vi "CV10.vi"() -> ()   [LabVIEW 2016]
uses:
  <vilib>/Analysis/baseanly.llb/Mean (DBL).vi
  <vilib>/DAQmx/read.llb/DAQmx Read (Analog 2D DBL NChan NSamp).vi
  <vilib>/DAQmx/create/channels.llb/DAQmx Create Channel (AI-Voltage-Basic).vi
  <vilib>/DAQmx/configure/timing.llb/DAQmx Timing (Sample Clock).vi
  <vilib>/DAQmx/miscellaneous.llb/DAQmx Fill In Error Info.vi
  <vilib>/imath/engines/lvmath2/RunTimeEngine/Managers/WorkSpace/UID Generator.vi
  <vilib>/imath/engines/lvmath2/RunTimeEngine/RunTimeType/NIMS_RunTimeType_From StrictType (excl LVString).vi
  <instcachedir>/0/NIMS_RunTimeType_From StrictType (excl LVString)_CEE1C65A8F1B491DB327E5E54E5E7674.lvgen/NIMS_RunTimeType_From StrictType (excl LVString)_CEE1C65A8F1B491DB327E5E54E5E7674_000.vi
  <vilib>/imath/engines/lvmath2/RunTimeEngine/LocalVariableDefStatement/MC_LocalVariableDefStatement_Display.vi
  <vilib>/imath/engines/lvmath2/RunTimeEngine/Managers/SymbolTable/Clear UID.vi
  <vilib>/imath/engines/lvmath2/RunTimeEngine/NodeEndStatement/NIMS_NodeEndStatement_Output.vi
  <instcachedir>/0/NIMS_NodeEndStatement_Output_53EC0D466D134D7ABD903AC30B43404B.lvgen/NIMS_NodeEndStatement_Output_53EC0D466D134D7ABD903AC30B43404B_009.vi
  <vilib>/imath/engines/lvmath2/RunTimeEngine/ErrorHandling/NIMS_Finalize Error.vi
  <vilib>/Analysis/NI_AALBase.lvlib
  <vilib>/imath/engines/lvmath2/RunTimeEngine/Managers/SymbolTable/NIMS_WorkSpace.lvlib
panel:
  out "Effective Sample Rate (Hz)":dbl=10.0
  in  "Display Length (s)":dbl=280.0 format="%#.3f"
  out "Time Step (ms)":dbl=100.0
  out "I-t":cluster{dbl[], dbl[]}(graph)
  in  "Samples to Average":i32=30000
  out "Elements in Queue":i32
  in  "Stop":bool
  in  "file path (use dialog), Create or Replace":path
  in  "Gain (mV/pA)":dbl=1.0
  out "I-V":cluster{dbl[], dbl[]}(graph)
  in  "Sampling Rate (Hz)":dbl=300000.0 format="%0.0f"
  in  "Voltage/Current Input Channels":tag="Dev1/ai0:1"
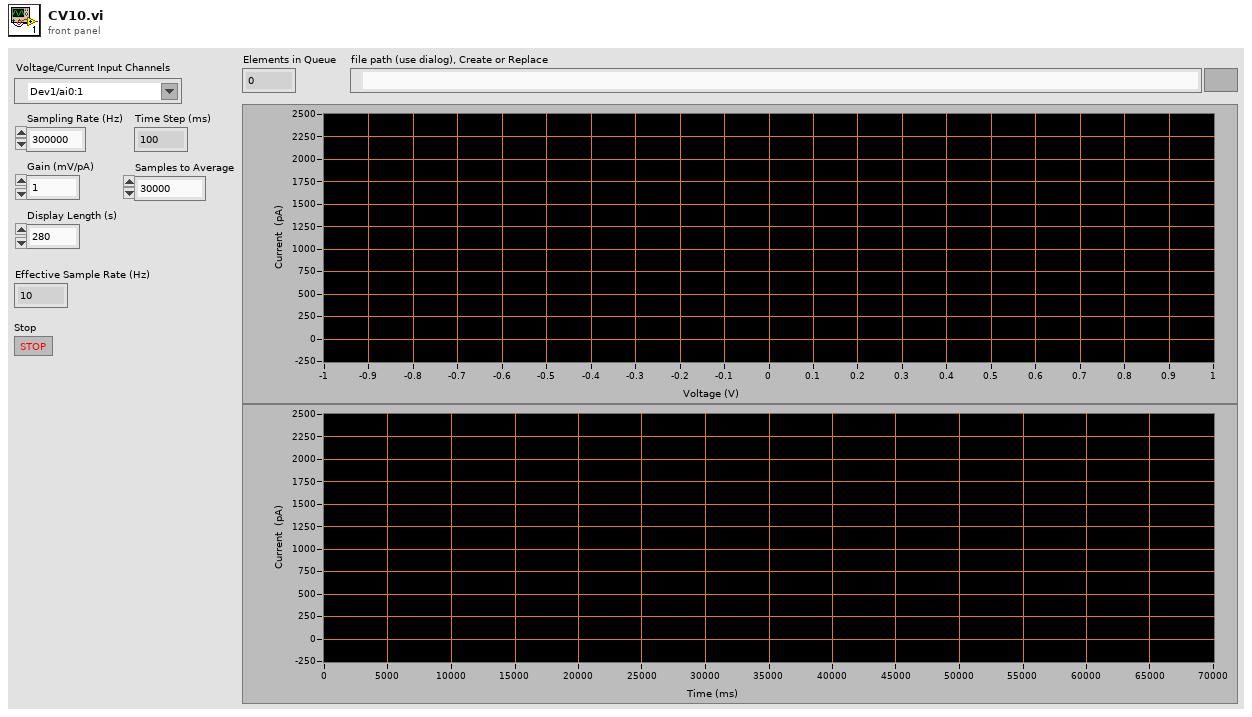
[diagram p1: front panel]
types:
  T1 = enum16{"open", "replace", "create", "open or create", "replace or create", "replace or create with confirmation"}
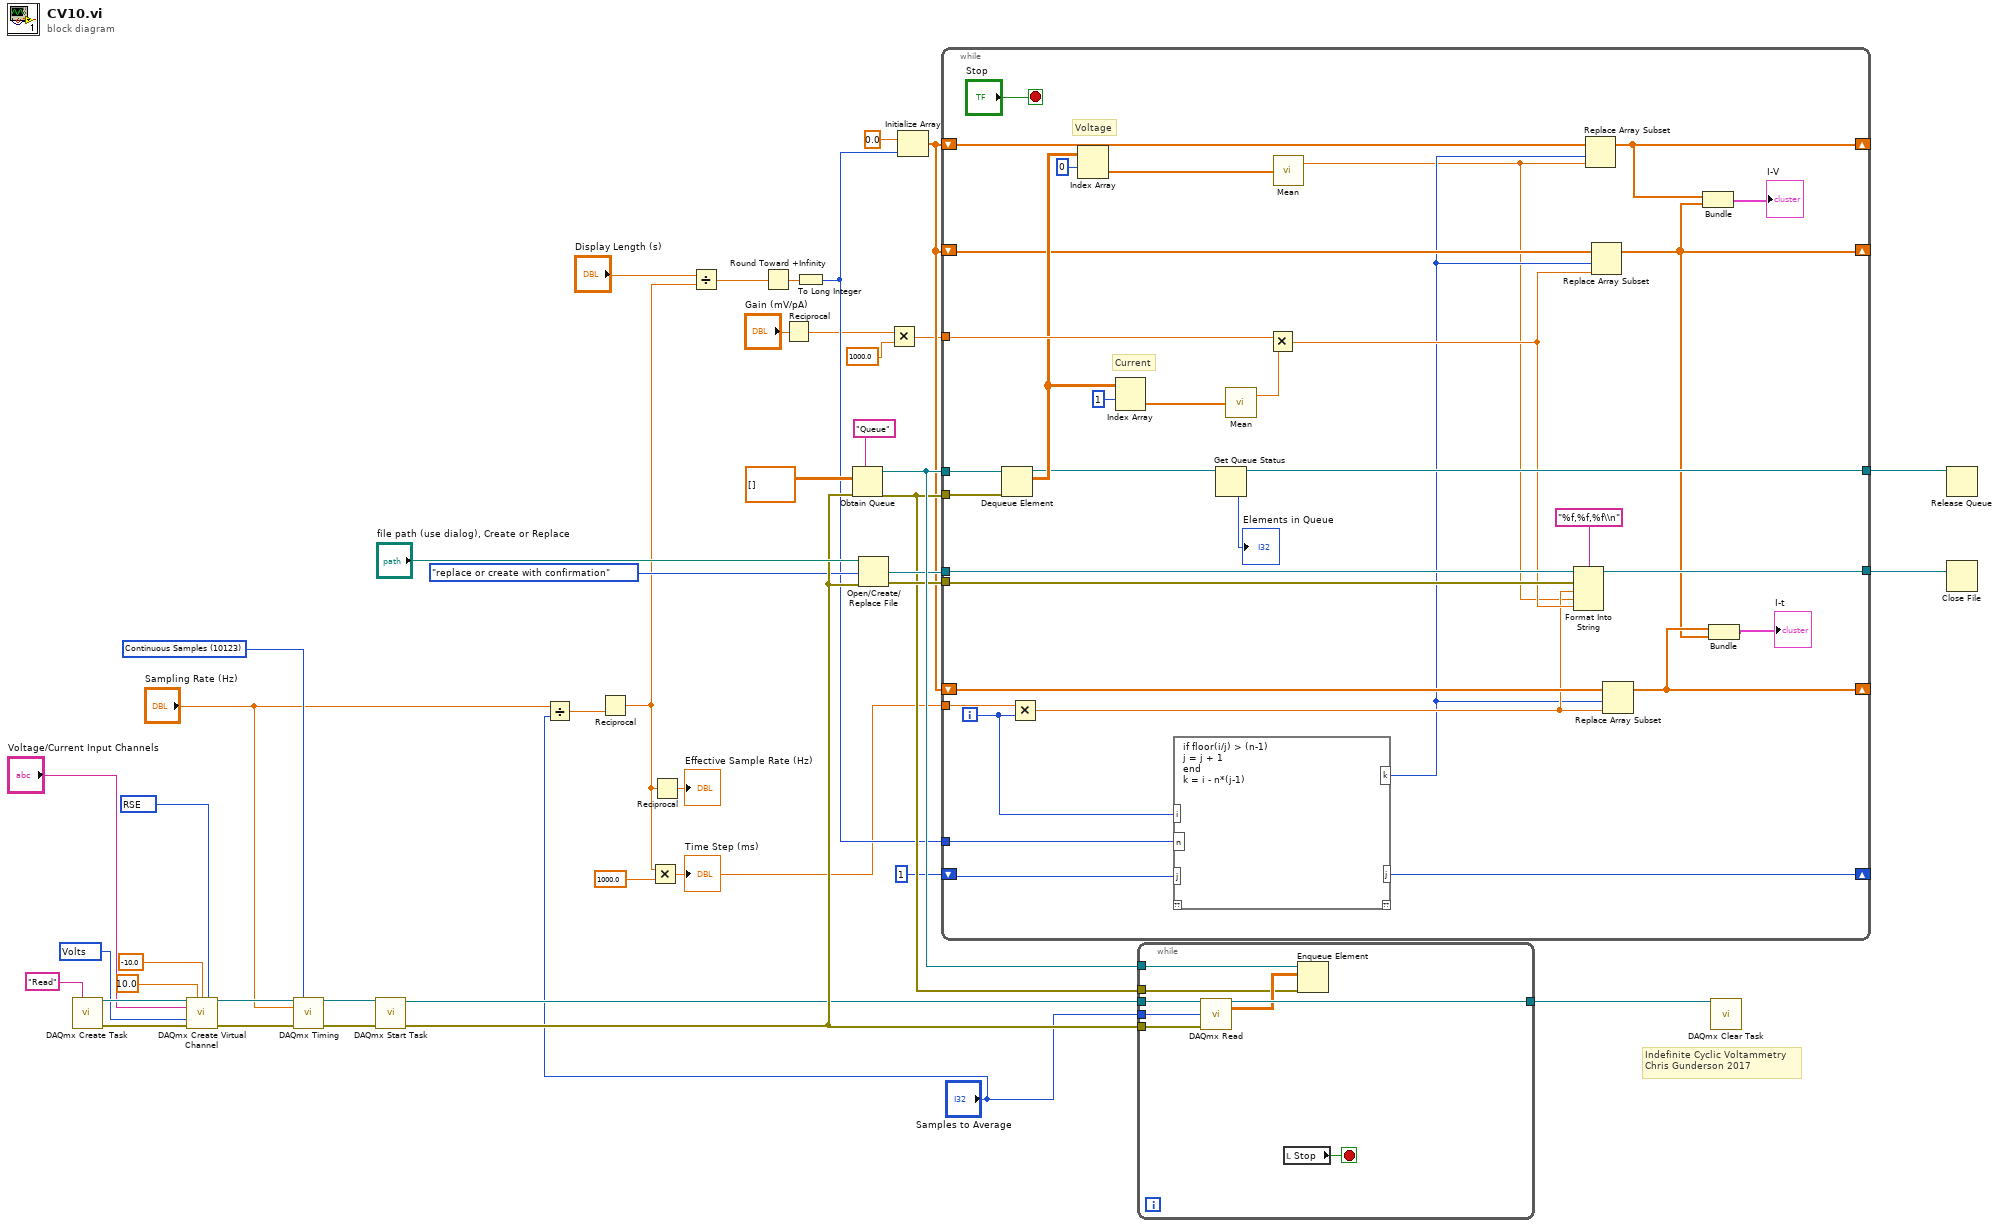
[diagram p0: block diagram]
diagram:
  w32 = 10123 items=["Finite Samples"=10178, "Continuous Samples"=10123, "Hardware Timed Single Point"=12522] ("sample mode")
  w35 = 10348 items=["Volts"=10348, "From Custom Scale"=10065] ("units")
  w36 = 10083 items=["Default"=-1, "RSE"=10083, "NRSE"=10078, "Differential"=10106, "Pseudodifferential"=12529] ("input terminal configuration")
  # "Indefinite Cyclic Voltammetry\nChris Gunderson 2017"
  n1 = call <vilib>:"DAQmx Create Task.vi"("new task name"="Read") -> ("task out"=w44:refnum<k21>, "error out"=w39:errorcluster)  [unwired: 13 in]
  n2 = call-poly <vilib>:"DAQmx Create Virtual Channel.vi"("task in"=w44, "maximum value"=10.0, "minimum value"=-10.0, "input terminal configuration"=w36, "physical channels"="Voltage/Current Input Channels", "units"=w35, "error in"=w39) -> ("task out"=w43:refnum<k21>, "error out"=w40:errorcluster)  [unwired: 7 in]
  n3 = call-poly <vilib>:"DAQmx Timing.vi"("task/channels in"=w43, "sample mode"=w32, "rate"="Sampling Rate (Hz)", "error in"=w40) -> ("task out"=w42:refnum<k21>, "error out"=w41:errorcluster)  [unwired: 10 in]
  n4 = call <vilib>:"DAQmx Start Task.vi"("task/channels in"=w42, "error in"=w41) -> ("task out"=w26:refnum<k21>, "error out"=w27:errorcluster)  [unwired: 12 in]
  n5 = Divide(x="Sampling Rate (Hz)", y="Samples to Average") -> (x/y=w14:dbl)
  n6 = Reciprocal(x=w14) -> (1/x=w2:dbl)
  n7 = Multiply(x=w2, y=1000.0) -> (x*y=w1:dbl)
  "Time Step (ms)" <- w1
  n8 = Reciprocal(x=w2) -> (1/x=→"Effective Sample Rate (Hz)":dbl)
  n9 = Divide(x="Display Length (s)", y=w2) -> (x/y=w9:dbl)
  n10 = Round Toward +Infinity(x=w9) -> (ceil(x): smallest int >= x=w8:dbl)
  n11 = Reciprocal(x="Gain (mV/pA)") -> (1/x=w5:dbl)
  n12 = To Long Integer(number=w8) -> (32bit integer=w7:i32)
  n13 = Obtain Queue(name (unnamed)="Queue", element data type=dbl[][] [], error in (no error)=w27) -> (queue out=w24:refnum<queue>, error out=w20:errorcluster)  [unwired: 2 in, 1 out]
  n14 = Open/Create/Replace File(file path (use dialog)="file path (use dialog), Create or Replace", error in=w27, operation (0:open)=T1."replace or create with confirmation") -> (refnum out=w21:refnum<file>, error out=w23:errorcluster)  [unwired: 3 in, 1 out]
  n15 = Multiply(x=w5, y=1000.0) -> (x*y=w4:dbl)
  n16 = Initialize Array(0.0 ("element"), w7) -> (w12:dbl[])
  n17 = while {
    shift-right: [w49] -> _
    shift-left: w12 -> [w63]
    shift-right: [w50] -> _
    shift-left: w12 -> [w62]
    tunnel: w4 -> [w76]
    tunnel: w24 -> [w74]
    tunnel: w23 -> [w73]
    tunnel: [w72] -> w22
    tunnel: w21 -> [w71]
    tunnel: w20 -> [w69]
    tunnel: [w67] -> w19
    tunnel: w1 -> [w64]
    shift-right: [w53] -> _
    shift-left: w12 -> [w60]
    tunnel: w7 -> [w57]
    shift-right: [w55] -> _
    shift-left: 1 ("j") -> [w56]
    i -> [w58]
    stop <- "Stop" stop-if-true
    # "Current"
    # "Voltage"
    n18 = Dequeue Element(queue=w74, error in (no error)=w69) -> (queue out=w68:refnum<queue>, element=w70:dbl[][])  [unwired: 1 in, 2 out]
    n19 = Multiply(x=w64, y=w58) -> (x*y=w59:dbl)
    n20 = Index Array(array=w70, index (row)=0 ("disabled index (col)")) -> (element=w47:dbl[])  [unwired: 1 in]
    n21 = Index Array(array=w70, index (row)=1 ("disabled index (col)")) -> (element=w45:dbl[])  [unwired: 1 in]
    n22 = mathscript code="if floor(i/j) > (n-1)\nj = j + 1\nend\nk = i - n*(j-1)"("i"=w58, "n"=w57, "j"=w56) -> ("j"=w55:i32, "k"=w54:i32)  [unwired: 1 in, 1 out]
    n23 = Get Queue Status(queue=w68) -> (queue out=w67:refnum<queue>, # elements in queue=→"Elements in Queue":i32)  [unwired: 2 in, 6 out]
    n24 = call-poly <vilib>:"Mean.vi"("X"=w45) -> ("mean"=w46:dbl)  [unwired: 1 out]
    n25 = Multiply(x=w76, y=w46) -> (x*y=w61:dbl)
    n26 = call-poly <vilib>:"Mean.vi"("X"=w47) -> ("mean"=w48:dbl)  [unwired: 1 out]
    n27 = Format Into String(format string="%f,%f,%f\\n", initial string=w71, error in=w73, w59, w48, w61) -> (resulting string=w72:refnum<file>)  [unwired: 1 out]
    n28 = Replace Array Subset(array=w63, new element=w48, index=w54) -> (w49:dbl[])
    n29 = Replace Array Subset(array=w62, new element=w61, index=w54) -> (w50:dbl[])
    n30 = Replace Array Subset(array=w60, new element=w59, index=w54) -> (w53:dbl[])
    n31 = Bundle(w49, w50) -> (→"I-V":cluster{dbl[], dbl[]})  [unwired: 1 in]
    n32 = Bundle(w53, w50) -> (→"I-t":cluster{dbl[], dbl[]})  [unwired: 1 in]
  }
  n33 = while {
    tunnel: w24 -> [w162]
    tunnel: w27 -> [w166]
    tunnel: w26 -> [w165]
    tunnel: [w164] -> w25
    tunnel: w20 -> [w161]
    tunnel: "Samples to Average" -> [w159]
    stop <- w160 stop-if-true
    n34 = call-poly <vilib>:"DAQmx Read.vi"("task/channels in"=w165, "number of samples per channel"=w159, "error in"=w166) -> ("task out"=w164:refnum<k21>, "data"=w163:dbl[][])  [unwired: 10 in, 1 out]
    n35 = local read "Stop"() -> (w160:bool)
    n36 = Enqueue Element(queue=w162, element=w163, error in (no error)=w161) -> ()  [unwired: 1 in, 3 out]
  }
  n37 = call <vilib>:"DAQmx Clear Task.vi"("task in"=w25) -> ()  [unwired: 14 in, 1 out]
  n38 = Release Queue(queue=w19) -> ()  [unwired: 2 in, 3 out]
  n39 = Close File(refnum=w22) -> ()  [unwired: 1 in, 2 out]
